vi "AsignedUnasigned.vi"(5 "Days Open Phone Treshhold":dbl=0.01, 6 "AE/ELP?":bool, 7 "AE Groups":T1[](array[typedef])=[enum."AE-Germany", enum."AE-Poland", enum."AE-Switzerland", enum."AE-Czech Republic", enum."AE-Hungary", enum."AE-Romania", enum."AE-Slovakia", enum."AE-Slovenia"], 8 "error in (no error)":errorcluster, 11 "All SR In":T2[](array[typedef])) -> (0 "error out":errorcluster, 2 "Unassigned":T2[](array[typedef]), 3 "Assigned Out":T2[](array[typedef]))   [LabVIEW 2017, in "Client.lvlib" / "ParserSorter.lvlib"]
doc: "Check If Days Open > 0,1 and calculate Score based on Prio specific Base Values"
uses:
  ParserSorter.lvlib
  TypeDefs/SRData.ctl
  TypeDefs/AEGroup.ctl
  TypeDefs/SRStatus.ctl
  TypeDefs/SRLevel.ctl
  TypeDefs/SRType.ctl
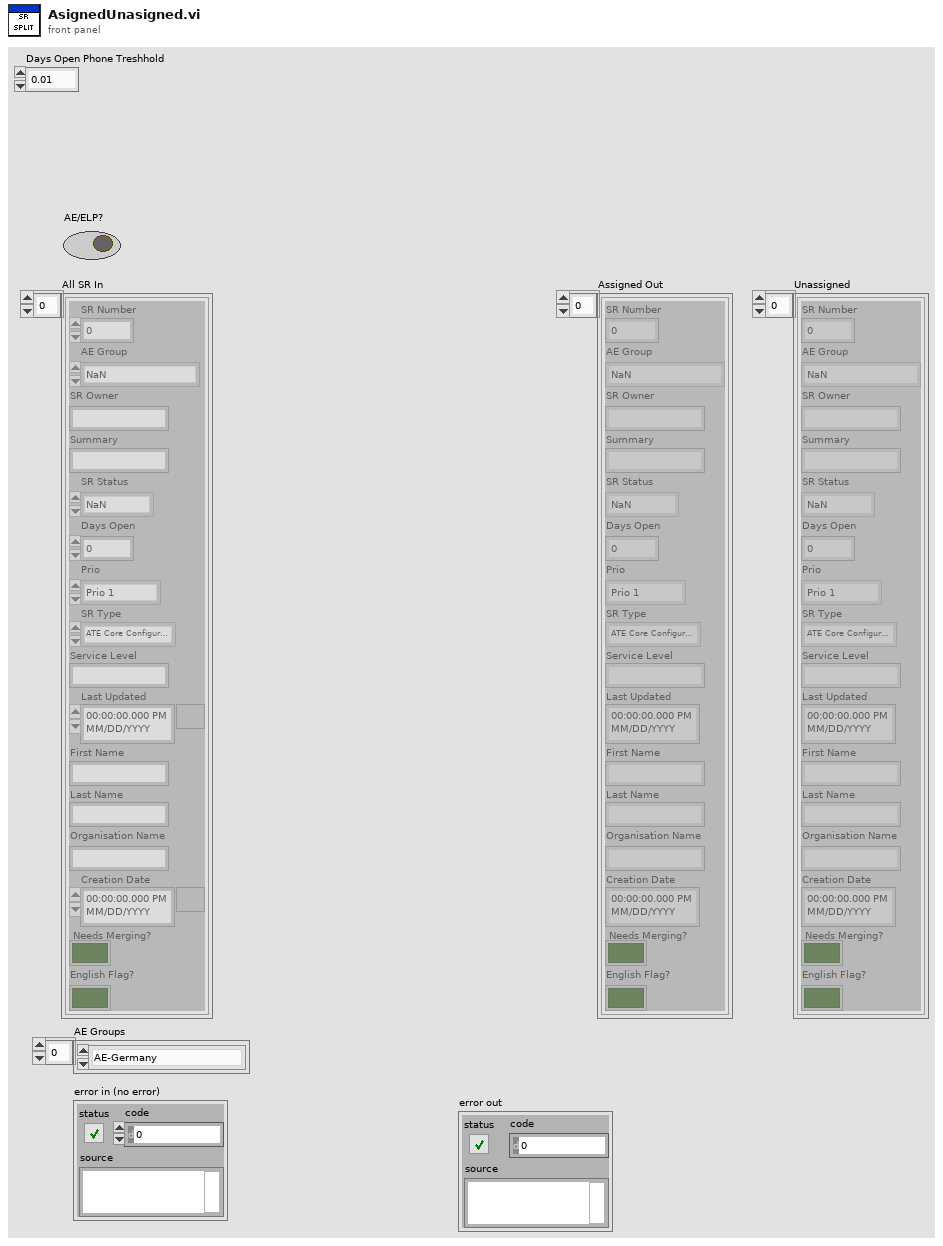
[diagram p1: front panel]
types:
  T1 = typedef "Client.lvlib/ParserSorter.lvlib/AEGroup.ctl" = enum32{"NaN", "AE-Germany", "AE-Poland", "AE-Switzerland", "AE-Czech Republic", "AE-Hungary", "AE-Romania", "AE-Slovakia", "AE-Slovenia"}
  T2 = typedef "Client.lvlib/ParserSorter.lvlib/SRData.ctl" = cluster{"SR Number":i64, "AE Group":T1, "SR Owner":string, "Summary":string, "SR Status":T3, "Days Open":dbl, "Prio":T4, "SR Type":T5, "Service Level":string, "Last Updated":timestamp, "First Name":string, "Last Name":string, "Organisation Name":string, "Creation Date":timestamp, "Needs Merging?":bool, "English Flag?":bool}
  T3 = typedef "Client.lvlib/ParserSorter.lvlib/SRStatus.ctl" = enum32{"NaN", "Caller Abandoned", "Created in Error", "Declined to Purchase Support", "Expired", "Forum Resolved AE", "Forum Resolved Customer", "IN WORK", "IN WORK Collab with AES", "IN WORK Collab with PSE", "IN WORK Collab with SE", "IN WORK Escalation", "IN WORK Customer Added Note", "Open", "Potentially Resolved", "POC Resolved", "Resolved", "RMA Waiting on Customer", "RMA Open", "RMA In Progress", "RMA Closed - DOA", "RMA Closed", "RMA Approved for Return", "Project Complete", "Presumed Resolved", "IN WORK Wait on Customer"}
  T4 = typedef "Client.lvlib/ParserSorter.lvlib/SRLevel.ctl" = enum16{"Prio 1", "Prio 2", "Prio 3", "Prio 4"}
  T5 = typedef "Client.lvlib/ParserSorter.lvlib/SRType.ctl" = enum32{"NaN", "ATE Core Configurations (BYOATE)", "Activation", "BioBench", "CAN", "CM C Series", "Calibration", "Consulting Services", "CounterTimer", "DAQExpress", "DASYLab", "DIAdem", "DMM", "DSA HW", "Digital_IO", "FIRST (NIC Only)", "FieldBus", "FieldPoint", "Functional Savety", "GATI", "GPIB", "HMI and Industrial PCs", "HiQ", "HighSpeedDigital_IO", "IMAQ", "IOTech Vibration", "Industrial Communications", "InsightCM", "LV", "LV CD&Sim", "LV Comms", "LV Controls Add-Ons", "LV Embedded", "LV MathScript RT", "LV NXG", "LV NXT", "LVDSC", "LVFPGA", "LVPDA and LV Touch Panel", "LVRT", "LabWindows_CVI", "Lookout", "MATRIXx", "MStudioDotNet", "MStudioVisualBasic", "MStudioVisualC", "Measure (Legacy)", "Motion", "MultifunctionDAQ", "Multimedia Test HW/SW", "Multisim (EWB)", "NI Update Service", "OPC Servers", "Optical (OSI)", "PXI Controllers, Chassis, MXI", "PXI Timing and Sync", "Power Supplies and SMUs", "Powertrain Controls", "RAID", "RF", "RF Software", "RIO", "SC Express", "SCC", "SCXI", "SPEEDY-33 (Hyperception)", "STS", "ScopeDigitizers", "Serial", "Signal Sources", "SignalCondOther", "SignalExpress", "Software Defined Intruments", "Sound and Vibration SW", "Switch Executive", "Switches", "TestStand", "USRP", "Ultiboard (EWB)", "VBench", "VI Logger", "VXI_MXI", "VeriStand", "VisionSW", "VolumeLicenseMgr", "WSN", "Web UI Builder", "myRIO"}
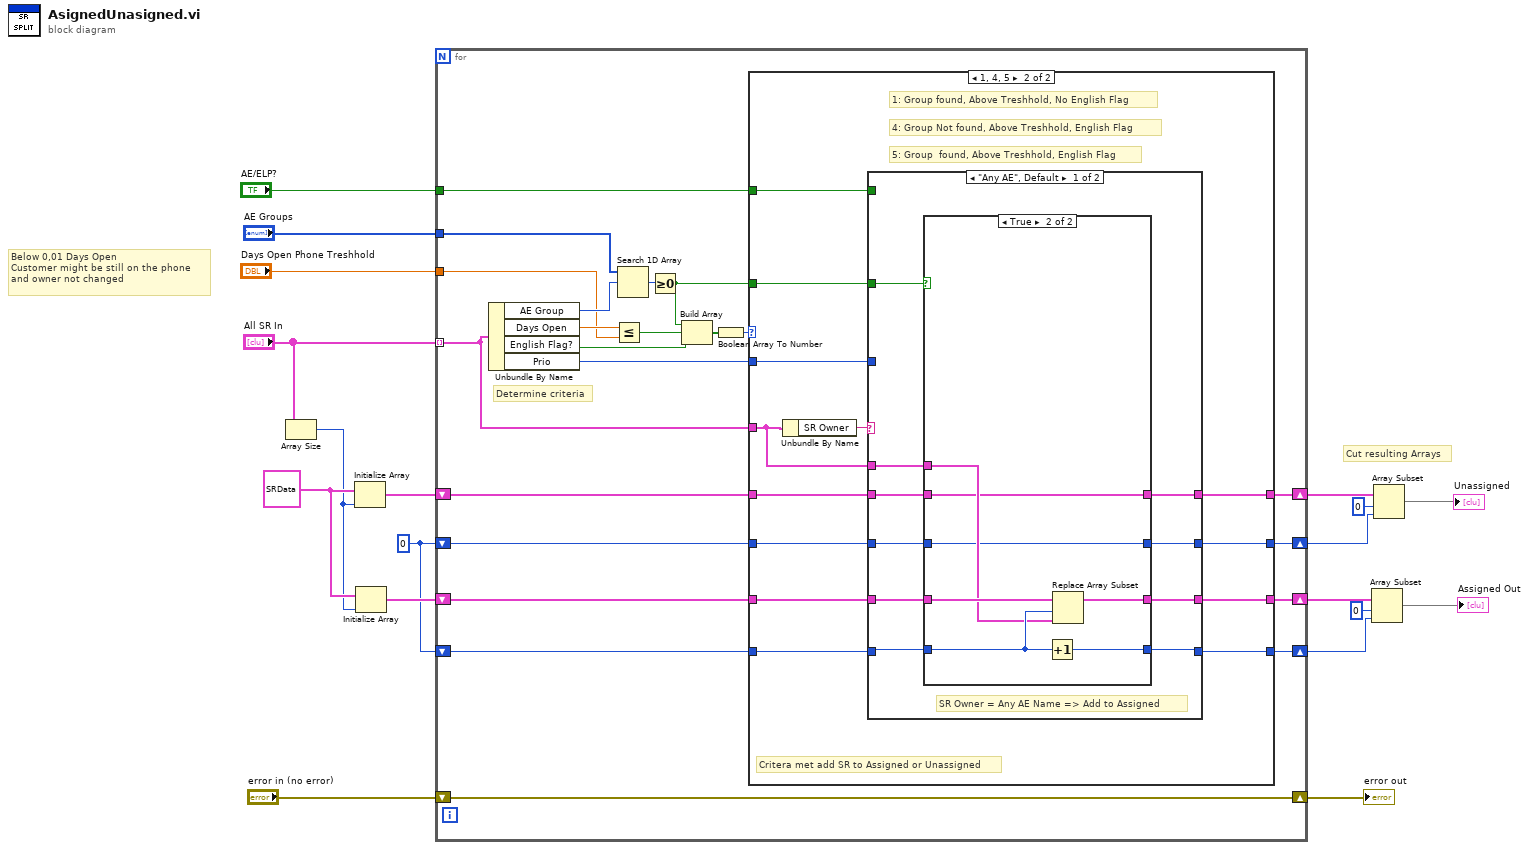
[diagram p0: block diagram]
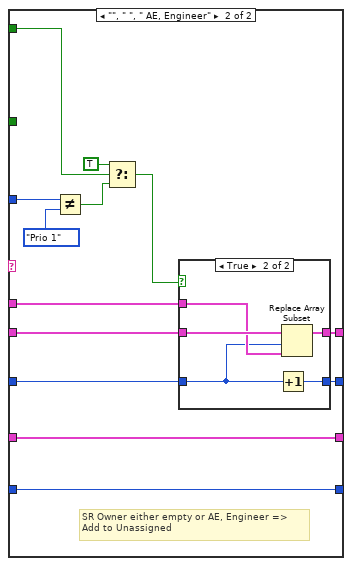
[diagram p4: hidden frame]
diagram:
  w12 = 0 ("size(s)")
  w16 = T2 {"SR Number"=0, "AE Group"=enum."NaN", "SR Owner"="", "Summary"="", "SR Status"=enum."NaN", "Days Open"=0.0, "Prio"=enum."Prio 1", "SR Type"=enum."ATE Core Configurations (BYOATE)", "Service Level"="", "Last Updated"=timestamp(0 s since 1904-01-01), "First Name"="", "Last Name"="", "Organisation Name"="", "Creation Date"=timestamp(0 s since 1904-01-01), "Needs Merging?"=FALSE, "English Flag?"=FALSE} ("SR Number")
  # "Below 0,01 Days Open\nCustomer might be still on the phone\nand owner not changed"
  # "Cut resulting Arrays"
  n1 = Array Size(array="All SR In") -> (size(s)=w15:i32)
  n2 = Initialize Array(w16, w15) -> (w13:T2[])
  n3 = Initialize Array(w16, w15) -> (w14:T2[])
  n4 = for {
    shift-right: [w41] -> w18
    shift-left: "error in (no error)" -> [w41]
    tunnel: "All SR In" -> [w38] mode=indexing
    shift-right: [w36] -> w7
    shift-left: w13 -> [w40]
    shift-right: [w35] -> w11
    shift-left: w14 -> [w34]
    shift-right: [w37] -> w4
    shift-left: w12 -> [w39]
    shift-right: [w33] -> w3
    shift-left: w12 -> [w32]
    tunnel: "Days Open Phone Treshhold" -> [w26]
    tunnel: "AE Groups" -> [w24]
    tunnel: "AE/ELP?" -> [w21]
    # "Determine criteria"
    n5 = Unbundle By Name(w38) -> ("AE Group"=w31:T1, "Days Open"=w27:dbl, "English Flag?"=w30:bool, "Prio"=w22:T4)
    n6 = Less Or Equal?(x=w27, y=w26) -> (x <= y?=w25:bool)
    n7 = Search 1D Array(1D array=w24, element=w31) -> (index of element=w23:i32)  [unwired: 1 in]
    n8 = Greater Or Equal To 0?(x=w23) -> (x >= 0?=w20:bool)
    n9 = Build Array(w20, w25, w30) -> (w28:bool[])
    n10 = Boolean Array To Number(Boolean array=w28) -> (number=w29:u32)
    n11 = case shown="1, 4, 5" w29 {
      tunnel: w40 -> [w45 w57]
      tunnel: w39 -> [w44 w55]
      tunnel: w38 -> [_ w49]
      tunnel: [w44 w51] -> w37
      tunnel: [w45 w50] -> w36
      tunnel: [w43 w52] -> w35
      tunnel: w34 -> [w43 w56]
      tunnel: [w42 w53] -> w33
      tunnel: w32 -> [w42 w54]
      tunnel: w22 -> [_ w48]
      tunnel: w21 -> [_ w47]
      tunnel: w20 -> [_ w46]
      frame 0, 2, 3, 6, 7, Default {
        # "6: Group Not found, Below Treshhold, No English Flag"
        # "7: Group  found, Below Treshhold,  English Flag"
        # "3: Group  found, Below Treshhold, No English Flag"
        # "2: Group Not found, Below Treshhold, No English Flag"
        # "Criteria not met, dont add to SR list"
      }
      frame 1, 4, 5 {
        # "5: Group  found, Above Treshhold, English Flag"
        # "4: Group Not found, Above Treshhold, English Flag"
        # "1: Group found, Above Treshhold, No English Flag"
        # "Critera met add SR to Assigned or Unassigned"
        n12 = Unbundle By Name(w49) -> ("SR Owner"=w58:string)
        n13 = case shown="\"Any AE\", Default" w58 {
          tunnel: w57 -> [w63 w92]
          tunnel: w55 -> [w61 w89]
          tunnel: w56 -> [w68 w86]
          tunnel: w54 -> [w65 w87]
          tunnel: [w62 w91] -> w50
          tunnel: w49 -> [w64 w90]
          tunnel: [w60 w88] -> w51
          tunnel: [w66 w87] -> w53
          tunnel: [w67 w86] -> w52
          tunnel: w48 -> [_ w82]
          tunnel: w47 -> [_ w85]
          tunnel: w46 -> [w59 _]
          frame "Any AE", Default {
            # "SR Owner = Any AE Name => Add to Assigned"
            n14 = case shown="True" w59 {
              tunnel: w68 -> [w70 w79]
              tunnel: [w70 w78] -> w67
              tunnel: [w69 w77] -> w66
              tunnel: w65 -> [w69 w76]
              tunnel: w64 -> [_ w75]
              tunnel: w63 -> [w72 w74]
              tunnel: [w72 w74] -> w62
              tunnel: w61 -> [w71 w73]
              tunnel: [w71 w73] -> w60
              frame False {
              }
              frame True {
                n15 = Increment(x=w76) -> (x+1=w77:i32)
                n16 = Replace Array Subset(array=w79, new element=w75, index=w76) -> (w78:T2[])
              }
            }
          }
          frame "", " ", " AE, Engineer" {
            # "SR Owner either empty or AE, Engineer => \nAdd to Unassigned"
            n17 = Not Equal?(x=w82, y=SRLevel."Prio 1") -> (x != y?=w80:bool)
            n18 = Select(t=TRUE, s=w85, f=w80) -> (s? t:f=w83:bool)
            n19 = case shown="True" w83 {
              tunnel: w92 -> [w94 w99]
              tunnel: [w94 w98] -> w91
              tunnel: w90 -> [_ w97]
              tunnel: w89 -> [w93 w96]
              tunnel: [w93 w95] -> w88
              frame False {
              }
              frame True {
                n20 = Increment(x=w96) -> (x+1=w95:i32)
                n21 = Replace Array Subset(array=w99, new element=w97, index=w96) -> (w98:T2[])
              }
            }
          }
        }
      }
    }
  }
  "error out" <- w18
  n22 = Array Subset(array=w11, index=0, length=w3) -> (→"Assigned Out":T2[])
  n23 = Array Subset(array=w7, index=0, length=w4) -> (→"Unassigned":T2[])
